vi "enum-case structure.vi"() -> ()   [LabVIEW 2015]
panel:
  in  "stop":bool
  out "Resultado":dbl
  in  "Dato B":dbl
  in  "Dato A":dbl
  in  "Enum":T1(ring)
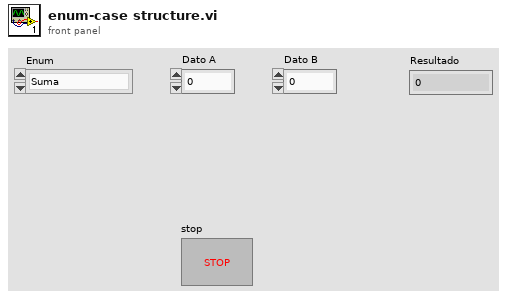
[diagram p1: front panel]
types:
  T1 = enum16{"Suma", "Resta", "Division", "Multiplicacion"}
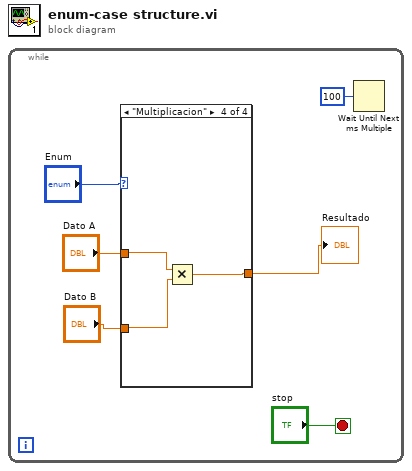
[diagram p0: block diagram]
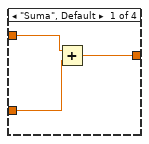
[diagram p2: hidden frame]
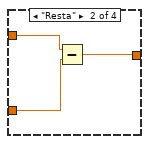
[diagram p3: hidden frame]
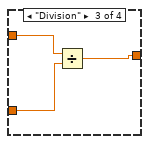
[diagram p4: hidden frame]
diagram:
  n1 = while {
    stop <- "stop" stop-if-true
    n2 = case shown="\"Multiplicacion\"" "Enum" {
      tunnel: "Dato A" -> [w9 w10 w15 w17]
      tunnel: "Dato B" -> [w8 w11 w14 w16]
      tunnel: [w7 w12 w13 w18] -> w2
      frame "Suma", Default {
        n3 = Add(x=w9, y=w8) -> (x+y=w7:dbl)
      }
      frame "Resta" {
        n4 = Subtract(x=w10, y=w11) -> (x-y=w12:dbl)
      }
      frame "Division" {
        n5 = Divide(x=w15, y=w14) -> (x/y=w13:dbl)
      }
      frame "Multiplicacion" {
        n6 = Multiply(x=w17, y=w16) -> (x*y=w18:dbl)
      }
    }
    "Resultado" <- w2
    n7 = Wait Until Next ms Multiple(millisecond multiple=u32 100) -> ()  [unwired: 1 out]
  }
